vi "Atheros RxGainCalibration.vi"(8 "error in (no error)":errorcluster, 9 "chainToCalibrate":u32, 10 "radioId":u32, 11 "_hResourceContext":u32) -> (0 "error out":errorcluster, 2 "function return":bool, 3 "_hResourceContext out":u32)   [LabVIEW 2013, in "QCAWLAN_DLL.lvlib"]
uses:
  QCAWLAN_DLL.lvlib
  QCAWLAN_DLL.dll
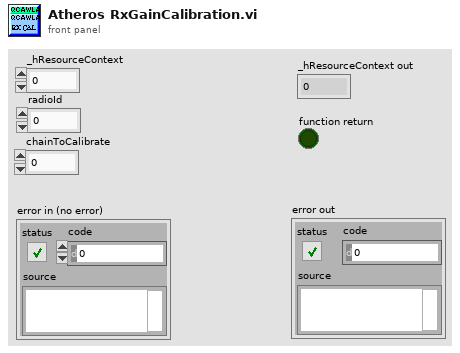
[diagram p1: front panel]
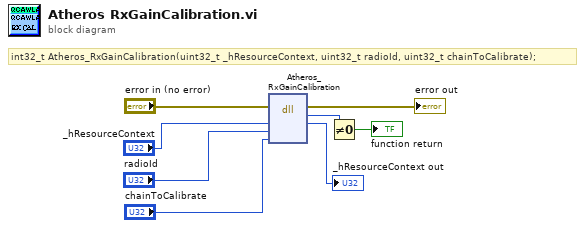
[diagram p0: block diagram]
diagram:
  # "int32_t Atheros_RxGainCalibration(uint32_t _hResourceContext, uint32_t radioId, uint32_t chainToCalibrate);"
  n1 = dll-call lib="C:/Connectivity Client - MIMO/PlugIn/QCAWLAN_DLL.dll" fn="Atheros_RxGainCalibration"(error in="error in (no error)", "_hResourceContext"="_hResourceContext", "radioId"="radioId", "chainToCalibrate"="chainToCalibrate") -> (error out=→"error out":errorcluster, "return type"=w7:i32, "_hResourceContext"=→"_hResourceContext out":u32)  [unwired: 4 in, 1 out]
  n2 = Not Equal To 0?(x=w7) -> (x != 0?=→"function return":bool)
